vi "Build_Read-Write Holding Registers.vi"(5 "write values":u16[](array[numeric]), 7 "write starting address":u16, 8 "error in (no error)":errorcluster, 9 "read quantity":u16, 10 "read starting address":u16) -> (0 "error out":errorcluster, 3 "MB_PDU":T1={"Function Code"=1, "Data"=[], "RTU_DataBytes"=0})   [LabVIEW 2012, in "MB Master.lvlib"]
doc: "Builds PDU for Read/Write Multiple Registers (function code 23)."
uses:
  MB Master.lvlib
  MB_PDU_Cluster.ctl
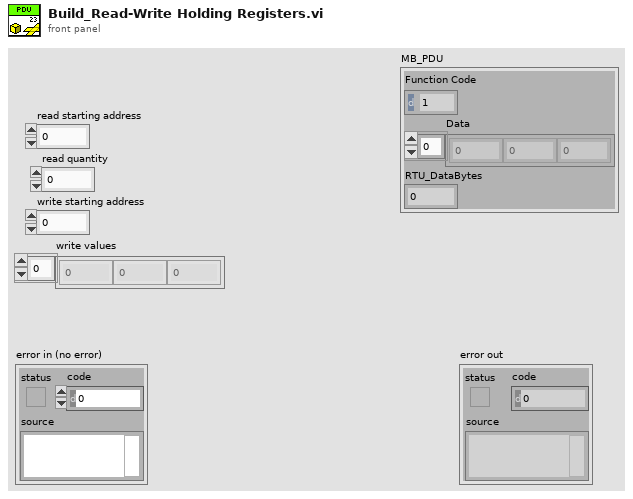
[diagram p1: front panel]
types:
  T1 = typedef "MB Master.lvlib/MB_PDU_Cluster.ctl" = cluster{"Function Code":u8, "Data":u8[], "RTU_DataBytes":i32}
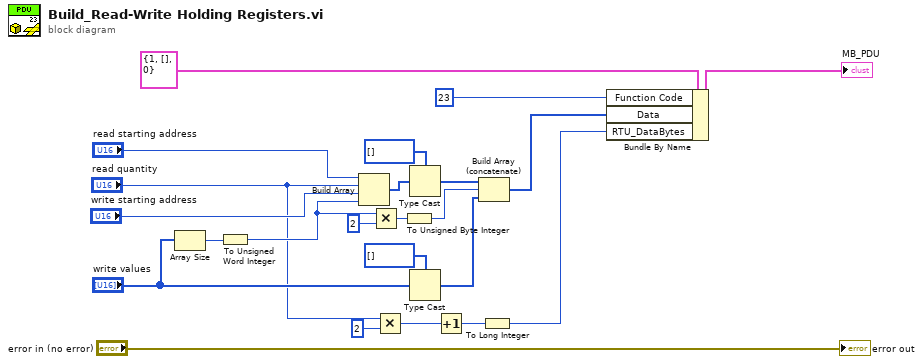
[diagram p0: block diagram]
diagram:
  n1 = Array Size(array="write values") -> (size(s)=w8:i32)
  n2 = To Unsigned Word Integer(number=w8) -> (unsigned 16bit integer=w6:u16)
  n3 = Build Array("read starting address", "read quantity", "write starting address", w6) -> (w23:u16[])
  n4 = Multiply(x=w6, y=u16 2) -> (x*y=w15:u16)
  n5 = Multiply(x="read quantity", y=u16 2) -> (x*y=w3:u16)
  n6 = To Unsigned Byte Integer(number=w15) -> (unsigned 8bit integer=w13:u8)
  n7 = Type Cast(type=u8[] [], x=w23) -> (*(type *) &x=w14:u8[])
  n8 = Type Cast(type=u8[] [], x="write values") -> (*(type *) &x=w11:u8[])
  n9 = Increment(x=w3) -> (x+1=w2:u16)
  n10 = Build Array (concatenate)(w14, w13, w11) -> (w10:u8[])
  n11 = To Long Integer(number=w2) -> (32bit integer=w1:i32)
  n12 = Bundle By Name(cluster=T1 {"Function Code"=1, "Data"=[], "RTU_DataBytes"=0} ("Modbus Serial New.lvlib:MB_PDU.lvclass"), "Function Code"=u8 23, "Data"=w10, "RTU_DataBytes"=w1) -> (→"MB_PDU":T1)
  "error out" <- "error in (no error)"
